vi "NetComm_CAN_GetStatus.vi"(8 "error in (no error)":errorcluster) -> (0 "error out":errorcluster, 1 "Transmit Error Count":u32, 2 "Receive Error Count":u32, 3 "Percent Bus Utilization":sgl, 4 "Bus Off Count":u32, 6 "Transmit FIFO Full Count":u32)   [LabVIEW 2017]
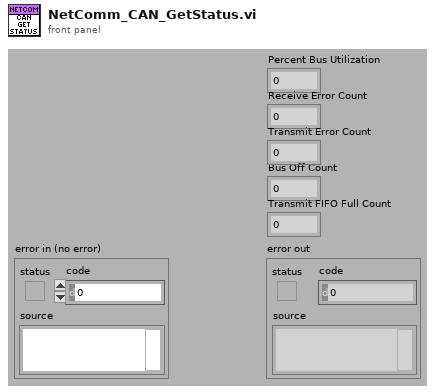
[diagram p1: front panel]
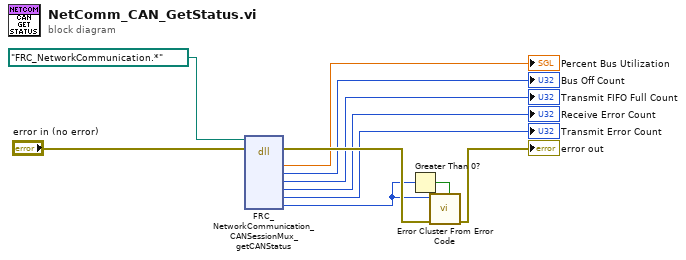
[diagram p0: block diagram]
diagram:
  n1 = dll-call lib="FRC_NetworkCommunication.*" fn="FRC_NetworkCommunication_CANSessionMux_getCANStatus"(path in=path "FRC_NetworkCommunication.*", error in="error in (no error)") -> (error out=w8:errorcluster, "percentBusUtilization"=→"Percent Bus Utilization":sgl, "busOffCount"=→"Bus Off Count":u32, "txFullCount"=→"Transmit FIFO Full Count":u32, "receiveErrorCount"=→"Receive Error Count":u32, "transmitErrorCount"=→"Transmit Error Count":u32, "status"=w6:i32)  [unwired: 8 in, 1 out]
  n2 = Greater Than 0?(x=w6) -> (x > 0?=w7:bool)
  n3 = call <vilib>:"Error Cluster From Error Code.vi"("is warning? (False)"=w7, "error in (no error)"=w8, "error code (0)"=w6) -> ("error out"=→"error out":errorcluster)  [unwired: 1 in, 5 out]
